vi "LRC-发送校验.vi"(11 "净数据":string) -> (3 "完整输出":string)   [LabVIEW 2013]
panel:
  out "十六进制整型字符串":string
  out "LRC":string
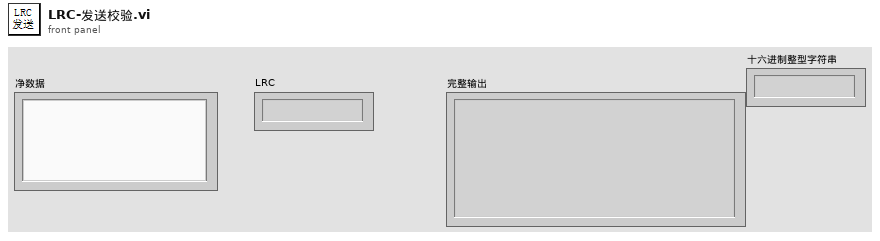
[diagram p1: front panel]
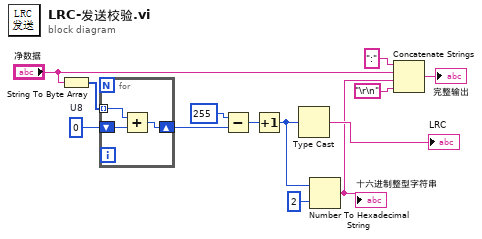
[diagram p0: block diagram]
diagram:
  w10 = u8 0  # U8
  n1 = String To Byte Array(string="净数据") -> (unsigned byte array=w5:u8[])
  n2 = for {
    shift-right: [w16] -> w6
    shift-left: w10 -> [w15]
    tunnel: w5 -> [w14] mode=indexing
    n3 = Add(x=w14, y=w15) -> (x+y=w16:u8)
  }
  n4 = Subtract(x=u8 255 ("无符号16位整型"), y=w6) -> (x-y=w7:u8)
  n5 = Increment(x=w7) -> (x+1=w4:u8)
  n6 = Type Cast(x=w4) -> (*(type *) &x=→"LRC":string)  [unwired: 1 in]
  n7 = Number To Hexadecimal String(1:i16 2 ("宽度(-)"), 2:w4) -> (0:w2:string)
  "十六进制整型字符串" <- w2
  n8 = Concatenate Strings(":", "净数据", w2, "\r\n") -> (→"完整输出":string)
